vi "Timed JSON Variant Tools.vi"() -> ()   [LabVIEW 2011]
doc: "Demonstrates the use of the Variant JSON VIs for converting to and from a complex cluster."
uses:
  JSON Value/Set from JSON string.vi
  Variant JSON/Variant to JSON.vi
  JSON Value/Get as JSON string (pretty).vi
  Variant JSON/Get as Variant.vi
  JSON Value/JSON Value.lvclass
  Get Polymorphic/JSON GetSet.lvlib
  Variant JSON/Variant JSON.lvlib
panel:
  out "Time":dbl format="%#_6p"
  out "error out":errorcluster
  out "Variant after setting":variant
  out "Cluster after setting":T1={"T1"=0.0, "Nest"={"NestNest"={"A"="", "Complex"=0.0+0.0i, "C"=0.0}, "Enum"=enum."AAA"}, "Test Array"=[], "Boolean 1"=FALSE, "T2"="", "Boolean 2"=FALSE, "Time Stamp"=timestamp(0 s since 1904-01-01), "Non JSON valid numerics"=0.0, "NAN"=0.0, "TTT"=0.0, "waveform"={"t0"=timestamp(0 s since 1904-01-01), "dt"=1.0, "Y"=[]}, "Test Array 2D"=[], "String Array"=[["", "", ""]], "Path"=path "", "App Refnum"=refnum}
  in  "Cluster to set":T1={"T1"=0.0, "Nest"={"NestNest"={"A"="", "Complex"=0.0+0.0i, "C"=0.0}, "Enum"=enum."AAA"}, "Test Array"=[], "Boolean 1"=FALSE, "T2"="", "Boolean 2"=FALSE, "Time Stamp"=timestamp(0 s since 1904-01-01), "Non JSON valid numerics"=0.0, "NAN"=0.0, "TTT"=0.0, "waveform"={"t0"=timestamp(0 s since 1904-01-01), "dt"=1.0, "Y"=[]}, "Test Array 2D"=[], "String Array"=[["", "", ""]], "Path"=path "", "App Refnum"=refnum}
  in  "Creation cluster":T2={"T2"="Test \"quote\",\nand newline.", "Nest"={"Enum"=enum."CCC (with a space)", "NestNest"={"A"=34.0, "Complex"=2.0+3.1i, "C"="1.23 string"}}, "Test Array"=[456.789, 2.0, 3.0], "Boolean 1"=TRUE, "T1"=456.789, "Boolean 2"="true (a string)", "Time Stamp"=timestamp(3434102896.3125 s since 1904-01-01), "Extra item"="test2", "Non JSON valid numerics"=inf, "NAN"=nan, "TTT"="any non number", "waveform"={"t0"=timestamp(3436250625 s since 1904-01-01), "dt"=1.0, "Y"=[23.0, 34.0]}, "Test Array 2D"=[[1.0, 2.0], [3.0, 4.0], [5.0, 6.0], [7.0, 8.0]], "String Array"=[["one", "number 2", "three"], ["1one", "two", "3"]], "Path"=path "c:/temp123.txt", "App Refnum"=refnum}
  out "JSON String created":string
  # "see diagram"
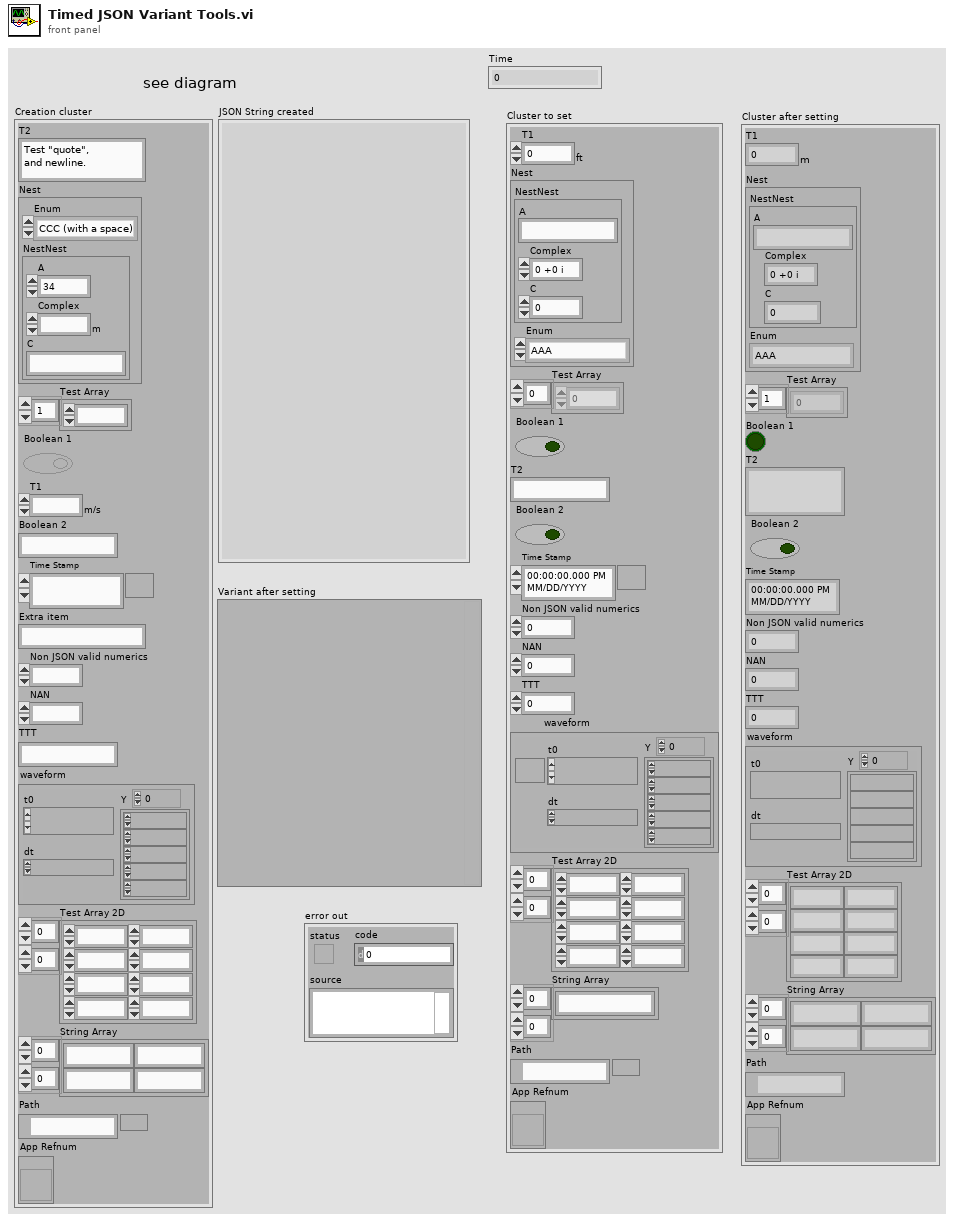
[diagram p1: front panel]
types:
  T1 = cluster{"T1":dbl[unit], "Nest":cluster{"NestNest":cluster{"A":string, "Complex":cdb, "C":dbl}, "Enum":enum16{"AAA", "BBB", "CCC (with a space)"}}, "Test Array":dbl[], "Boolean 1":bool, "T2":string, "Boolean 2":bool, "Time Stamp":timestamp, "Non JSON valid numerics":dbl, "NAN":dbl, "TTT":dbl, "waveform":waveform(dbl), "Test Array 2D":dbl[][], "String Array":string[][], "Path":path, "App Refnum":refnum<vi>}
  T2 = cluster{"T2":string, "Nest":cluster{"Enum":enum16{"AAA", "BBB", "CCC (with a space)"}, "NestNest":cluster{"A":dbl, "Complex":cdb[unit], "C":string}}, "Test Array":dbl[], "Boolean 1":bool, "T1":dbl[unit], "Boolean 2":string, "Time Stamp":timestamp, "Extra item":string, "Non JSON valid numerics":dbl, "NAN":dbl, "TTT":string, "waveform":waveform(dbl), "Test Array 2D":dbl[][], "String Array":string[][], "Path":path, "App Refnum":refnum<vi>}
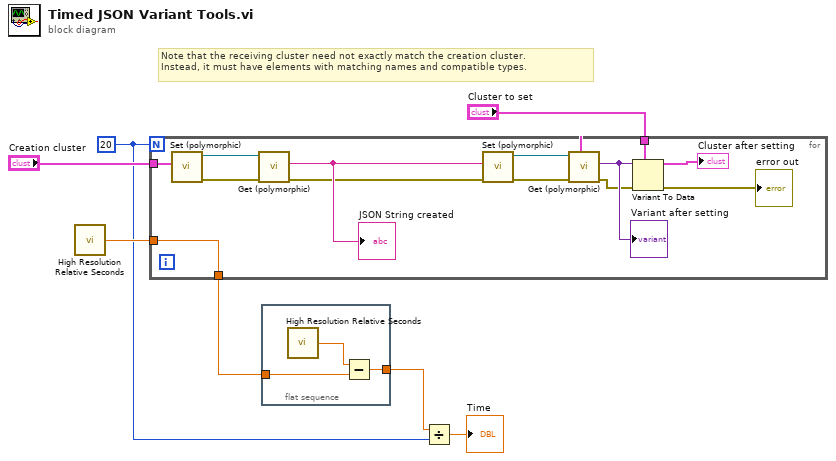
[diagram p0: block diagram]
diagram:
  w2 = 20
  # "Note that the receiving cluster need not exactly match the creation cluster.\nInstead, it must have elements with matching names and compatible types."
  n1 = call <vilib>:"High Resolution Relative Seconds.vi"() -> ("relative seconds"=w5:dbl)
  n2 = for {
    N: w2 -> [_]
    tunnel: "Creation cluster" -> [w12]
    tunnel: "Cluster to set" -> [w10]
    tunnel: w5 -> [w8]
    tunnel: [w8] -> w4
    n3 = call-poly "Set (polymorphic).vi"("Variant"=w12) -> ("error out"=w15:errorcluster, "JSON Value out"=w20:refnum<class "JSON Value.lvclass">)  [unwired: 9 in]
    n4 = call-poly "Get (polymorphic).vi"("error in (no error)"=w15, "JSON Value in"=w20) -> ("error out"=w14:errorcluster, "String"=w16:string)  [unwired: 8 in]
    "JSON String created" <- w16
    n5 = call-poly "Set (polymorphic).vi"("error in (no error)"=w14, "JSON stream"=w16) -> ("error out"=w11:errorcluster, "JSON Value out"=w13:refnum<class "JSON Value.lvclass">)  [unwired: 7 in, 1 out]
    n6 = call-poly "Get (polymorphic).vi"("Variant (Data Type)"=w10, "error in (no error)"=w11, "JSON in"=w13) -> ("error out"=w17:errorcluster, "Variant out"=w19:variant)  [unwired: 6 in, 1 out]
    "Variant after setting" <- w19
    n7 = Variant To Data(error in=w17, type=w10, Variant=w19) -> (data=→"Cluster after setting":T1, error out=→"error out":errorcluster)
  }
  n8 = flat-sequence {
    tunnel: w4 -> [w22]
    tunnel: [w21] -> w3
    frame #0 {
      n9 = call <vilib>:"High Resolution Relative Seconds.vi"() -> ("relative seconds"=w23:dbl)
      n10 = Subtract(x=w23, y=w22) -> (x-y=w21:dbl)
    }
  }
  n11 = Divide(x=w3, y=w2) -> (x/y=→"Time":dbl)
